vi "Choreo_SwerveSample_GetChassisSpeeds.vi"(11 "ChoreoSwerveSample":T2) -> (3 "ChassisSpeeds":T1 {"vOmega" format="%10.3f"; "vY" format="%10.3f"; "vX" format="%10.3f"})   [LabVIEW 2019, in "ChoreoLib.lvlib"]
doc: "Constructs a SwerveSample with the specified parameters.\n\n */\n\nInputs: \n - t - double - The timestamp of this sample, relative to the beginning of the trajectory.\n - x - double - The X position of the sample in meters.\n - y - double - The Y position of the sample in meters.\n - heading - double - The heading of the sample in radians, with 0 being in the +X direction.\n - vx - double - The velocity of the sample in the X direction in m/s.\n - vy - double - The velocity of the sample in the Y direction in m/s.\n - omega - double - The angular velocity of the sample in rad/s.\n - ax - double - The acceleration of the sample in the X direction in m/s².\n - ay - double - The acceleration of the sample in the Y direction in m/s².\n - alpha - double - The angular acceleration of the sample in rad/s².\n - moduleForcesX - double array - The force on each swerve module in the X direction in Newtons. Module forces appear in the following order: [FL, FR, BL, BR].\n - moduleForcesY - double array - The force on each swerve module in the Y direction in Newtons. Module forces appear in the following order: [FL, FR, BL, BR].\n\nOutputs:\n - ChoreoSwerveSample - cluster - Cluster containing sample data"
uses:
  TypeDef/ChoreoSwerveSample.ctl
  ChoreoLib.lvlib
  <vilib>/Rock Robotics/WPI/ThirdParty/JAS_Junk/TrajLib/Trajectory_Library.lvlib
  <vilib>/Rock Robotics/WPI/ThirdParty/JAS_Junk/TrajLib/TypeDef/CHASSIS_SPEEDS.ctl
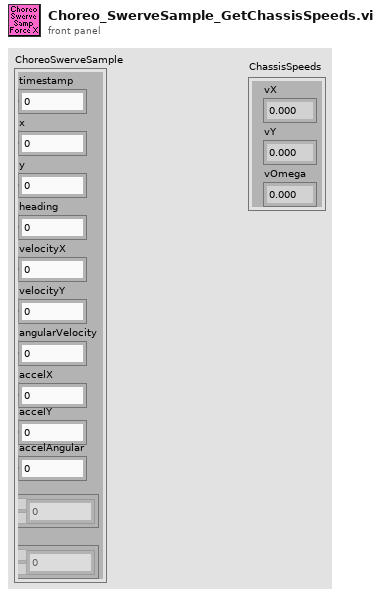
[diagram p1: front panel]
types:
  T1 = typedef "Trajectory_Library.lvlib/CHASSIS_SPEEDS.ctl" = cluster{"vX":dbl, "vY":dbl, "vOmega":dbl}
  T2 = typedef "ChoreoLib.lvlib/ChoreoSwerveSample.ctl" = cluster{"timestamp":dbl, "x":dbl, "y":dbl, "heading":dbl, "velocityX":dbl, "velocityY":dbl, "angularVelocity":dbl, "accelY":dbl, "accelX":dbl, "accelAngular":dbl, "forceX":dbl[], "forceY":dbl[]}
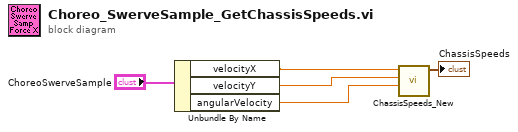
[diagram p0: block diagram]
diagram:
  n1 = Unbundle By Name("ChoreoSwerveSample") -> ("velocityX"=w4:dbl, "velocityY"=w3:dbl, "angularVelocity"=w2:dbl)
  n2 = call <vilib>:"ChassisSpeeds_New.vi"("vAngular"=w2, "vY"=w3, "vX"=w4) -> ("CHASSIS"=→"ChassisSpeeds":T1)  [unwired: 8 in]
